vi "Browse Variant_GetRef.vi"(8 "error in (no error)":errorcluster, 11 "VariantProbe.lvclass in":refnum<class "VariantTree__VP.lvclass">) -> (0 "error out":errorcluster, 2 "Tree Ref":refnum<vi>, 3 "VariantProbe.lvclass out":refnum<class "VariantTree__VP.lvclass">)   [LabVIEW 2011, in "VariantTree__VP.lvclass"]
uses:
  VariantTree__VP.lvclass
  VariantTree__VP.lvclass/VariantTree__VP.ctl
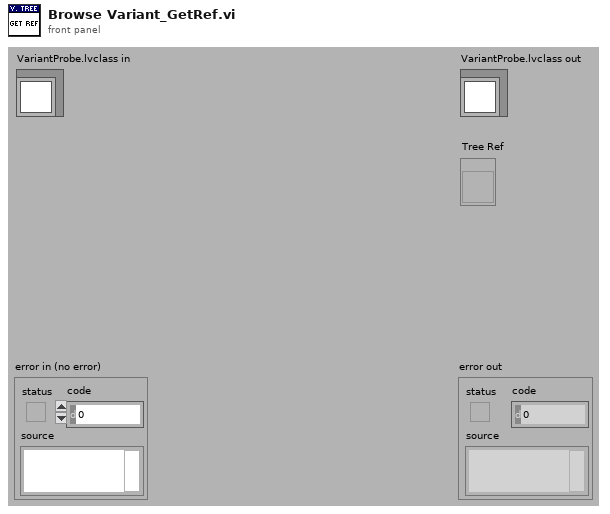
[diagram p1: front panel]
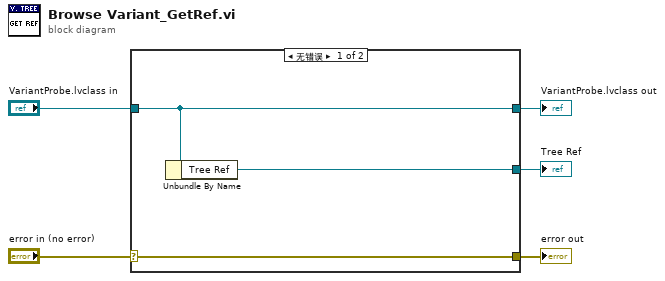
[diagram p0: block diagram]
diagram:
  n1 = case shown="无错误" "error in (no error)" {
    selector: "error in (no error)" -> [w8 w9]
    tunnel: [w8 w9] -> w4
    tunnel: [w7 w10] -> w2
    tunnel: "VariantProbe.lvclass in" -> [w7 w10]
    tunnel: [w6 _] -> w1
    frame No Error {
      n2 = Unbundle By Name(w7) -> ("Tree Ref"=w6:refnum<vi>)
    }
    frame Error {
    }
  }
  "error out" <- w4
  "VariantProbe.lvclass out" <- w2
  "Tree Ref" <- w1
